vi "KE622x -- 2182 -A Get Digital Filter Window.vi"(0 "622x Resource In":refnum<visa-resource-name>, 1 "Check For SCPI Errors? (T)":bool=TRUE, 11 "error in (no error)":errorcluster) -> (4 "622x Resource Out (dupl)":refnum<visa-resource-name>, 8 "Filter Window (%)":dbl=0.01 format="%#_13g", 15 "error out":errorcluster)   [LabVIEW 2013, in "Keithly user program.lvlib"]
uses:
  Keithly user program.lvlib
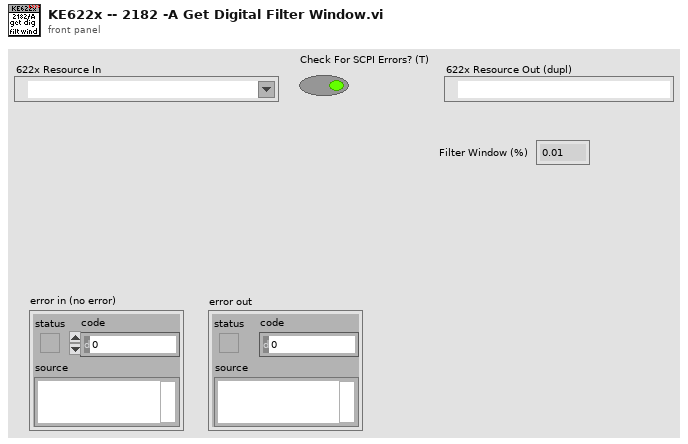
[diagram p1: front panel]
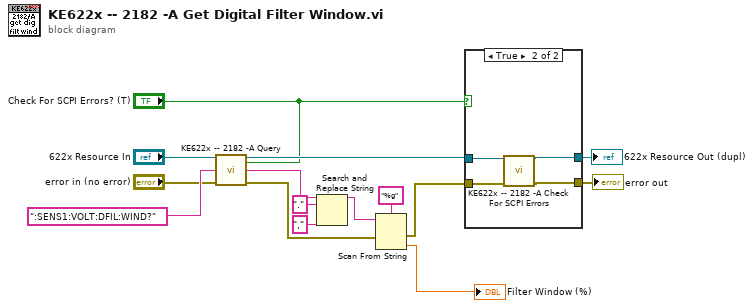
[diagram p0: block diagram]
diagram:
  n1 = call "KE622x -- 2182 -A Query.vi"("622x Resource In"="622x Resource In", "Check For SCPI Errors? (T)"="Check For SCPI Errors? (T)", "2182-A Write String"=":SENS1:VOLT:DFIL:WIND?", "error in (no error)"="error in (no error)") -> ("622x Resource Out (dupl)"=w10:refnum<visa-resource-name>, "2182-A Reponse String"=w4:string, "error out"=w5:errorcluster)  [unwired: 9 in]
  n2 = Search and Replace String(input string=w4, search string=".", replace string="," ("replace string (\"\")")) -> (result string=w3:string)  [unwired: 5 in, 3 out]
  n3 = Scan From String(format string="%g", input string=w3, error in=w5) -> (error out=w14:errorcluster, output 1=→"Filter Window (%)":dbl)  [unwired: 2 in, 2 out]
  n4 = case shown="True" "Check For SCPI Errors? (T)" {
    tunnel: w10 -> [w17 w21]
    tunnel: w14 -> [w16 w19]
    tunnel: [w17 w20] -> w13
    tunnel: [w16 w18] -> w12
    frame False {
    }
    frame True {
      n5 = call "KE622x -- 2182 -A Check For SCPI Errors.vi"("VISA Resource In"=w21, "error in (no error)"=w19) -> ("VISA Resource Out (dupl)"=w20:refnum<visa-resource-name>, "error out"=w18:errorcluster)  [unwired: 10 in, 2 out]
    }
  }
  "622x Resource Out (dupl)" <- w13
  "error out" <- w12
